vi "GetWebsocketInfo.vi"(5 "error in (no error)":errorcluster) -> (16 "Websocket Info":T1, 19 "error out":errorcluster)   [LabVIEW 2014, in "FrontPanelPublisher.lvlib" / "FrontPanelManager.lvclass"]
uses:
  FrontPanelManager.lvclass
  Controls/WebsocketInfo.ctl
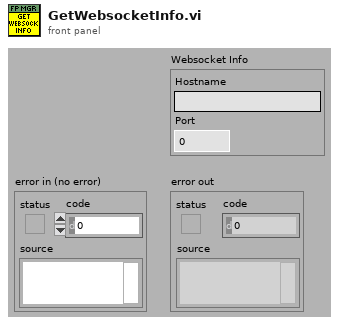
[diagram p1: front panel]
types:
  T1 = typedef "FrontPanelPublisher.lvlib/FrontPanelManager.lvclass/WebsocketInfo.ctl" = cluster{"Hostname":string, "Port":u16}
  T2 = typedef "FrontPanelPublisher.lvlib/FrontPanelManager.lvclass/ObjectAttributes.ctl" = cluster{"WebFrontPanels":refnum<class "WebFrontPanel.lvclass">[], "WFP Names":string[], "Root folder":path, "Websocket Info":T1}
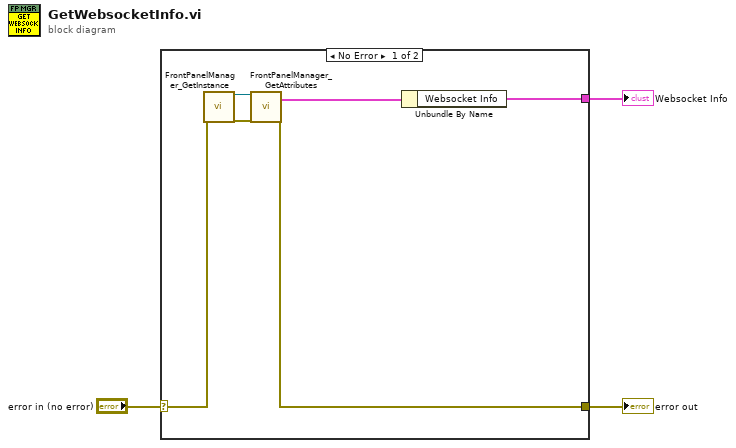
[diagram p0: block diagram]
diagram:
  n1 = case shown="No Error" "error in (no error)" {
    selector: "error in (no error)" -> [w5 w10]
    tunnel: [w8 w10] -> w2
    tunnel: [w7 _] -> w1
    frame No Error {
      n2 = call "FrontPanelManager_GetInstance.vi"("error in (no error)"=w5) -> ("reference out"=w6:refnum<class "FrontPanelManager.lvclass">, "error out"=w4:errorcluster)  [unwired: 14 in, 3 out]
      n3 = call "FrontPanelManager_GetAttributes.vi"("reference in"=w6, "error in (no error)"=w4) -> ("Data"=w9:T2, "error out"=w8:errorcluster)  [unwired: 14 in, 2 out]
      n4 = Unbundle By Name(w9) -> ("Websocket Info"=w7:T1)
    }
    frame Error {
    }
  }
  "error out" <- w2
  "Websocket Info" <- w1
